vi "Update Scaling Information.vi"(0 "Plugin_UI in":refnum<class "Plugin_UI.lvclass">, 11 "error in (no error)":errorcluster) -> (4 "Plugin_UI out":refnum<class "Plugin_UI.lvclass">, 15 "error out":errorcluster)   [LabVIEW 2020, in "Plugin.lvlib" / "Plugin_UI.lvclass"]
doc: "When the plugin is activated, read the latest scaling information from Module configuration and update it in the corresponding Channel object."
uses:
  Plugin_UI.lvclass
  C:/SVN_LabSys/labsys_lvcode/LabSys_SourceCode/builds/Libraries/LabSys Framework.lvlibp/Configurable Data Node/Configuration Interface/Configuration Interface.lvclass
  Plugin_UI.lvclass/Plugin_UI.ctl
  Read Input Channels[].vi
  Write Input Channels[].vi
  Channels/Input Channels/Input Channels.lvclass
  C:/SVN_LabSys/labsys_lvcode/LabSys_SourceCode/Plugin Template/Source/Code/Channels/Plugin_Channels.lvclass
  builds/Libraries/LabSys Framework.lvlibp/Configurable Data Node/Configuration Interface/Read Module Configuration.vi
  builds/Libraries/LabSys Framework.lvlibp/Configuration Storage/Module Configuration/Get Lookup Tables.vi
  builds/Libraries/LabSys Framework.lvlibp/Configuration Storage/Module Configuration/Get Scaling Functions.vi
  Write Lookup Tables.vi
  Write Scaling Functions.vi
  builds/Libraries/LabSys Framework.lvlibp/Configuration Storage/Module Configuration/Module Configuration.lvclass
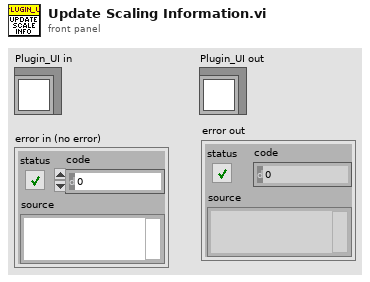
[diagram p1: front panel]
types:
  T1 = typedef "LabSys Framework.lvlibp/Configuration Storage.lvlib/Test Configuration.lvclass/Table Information.ctl" = cluster{"Name":string, "Lookup Table":dbl[][]}
  T2 = typedef "LabSys Framework.lvlibp/Configuration Storage.lvlib/Test Configuration.lvclass/Function Information.ctl" = cluster{"Name":string, "Expression":string, "Constants":T3[], "Test Data":dbl[][]}
  T3 = typedef "LabSys Framework.lvlibp/Configuration Storage.lvlib/Test Configuration.lvclass/Function Constant Value.ctl" = cluster{"Constant Name":string, "Value":dbl}
  T4 = typedef "LabSys Framework.lvlibp/Configuration Storage.lvlib/Test Configuration.lvclass/Channel Information.ctl" = cluster{"Channel Direction":T5, "Alias":string, "Refresh (ms)":dbl, "Scaling Information":T6, "Value Type":T8, "Subchannels":T9[], "Auxiliary Data":variant, "Group":i32}
  T5 = typedef "LabSys Framework.lvlibp/Configuration Storage.lvlib/Test Configuration.lvclass/Channel Directions.ctl" = enum8{"Module Input", "Module Output"}
  T6 = typedef "LabSys Framework.lvlibp/Configuration Storage.lvlib/Test Configuration.lvclass/Scaling Information.ctl" = cluster{"Active":bool, "Scaling Type":T7, "Output Minimum":dbl, "Output Maximum":dbl, "Raw Minimum":dbl, "Raw Maximum":dbl, "Output Unit":string, "Function":string, "Lookup Table":string}
  T7 = typedef "LabSys Framework.lvlibp/Configuration Storage.lvlib/Test Configuration.lvclass/Scaling Types.ctl" = enum8{"Linear", "Function", "Lookup Table"}
  T8 = typedef "Framework Base Library.lvlibp/Value Types.ctl" = enum8{"Unknown", "double", "double array", "Waveform", "DigWaveform", "Boolean", "Decimal", "String", "Db2Message", "Byte Array", "Unsigned Decimal"}
  T9 = typedef "LabSys Framework.lvlibp/Configuration Storage.lvlib/Test Configuration.lvclass/Subchannel Information.ctl" = cluster{"Alias":string, "Start Bit":u32, "Bit Length":u32, "Value Type":T8, "Auxiliary Data":variant}
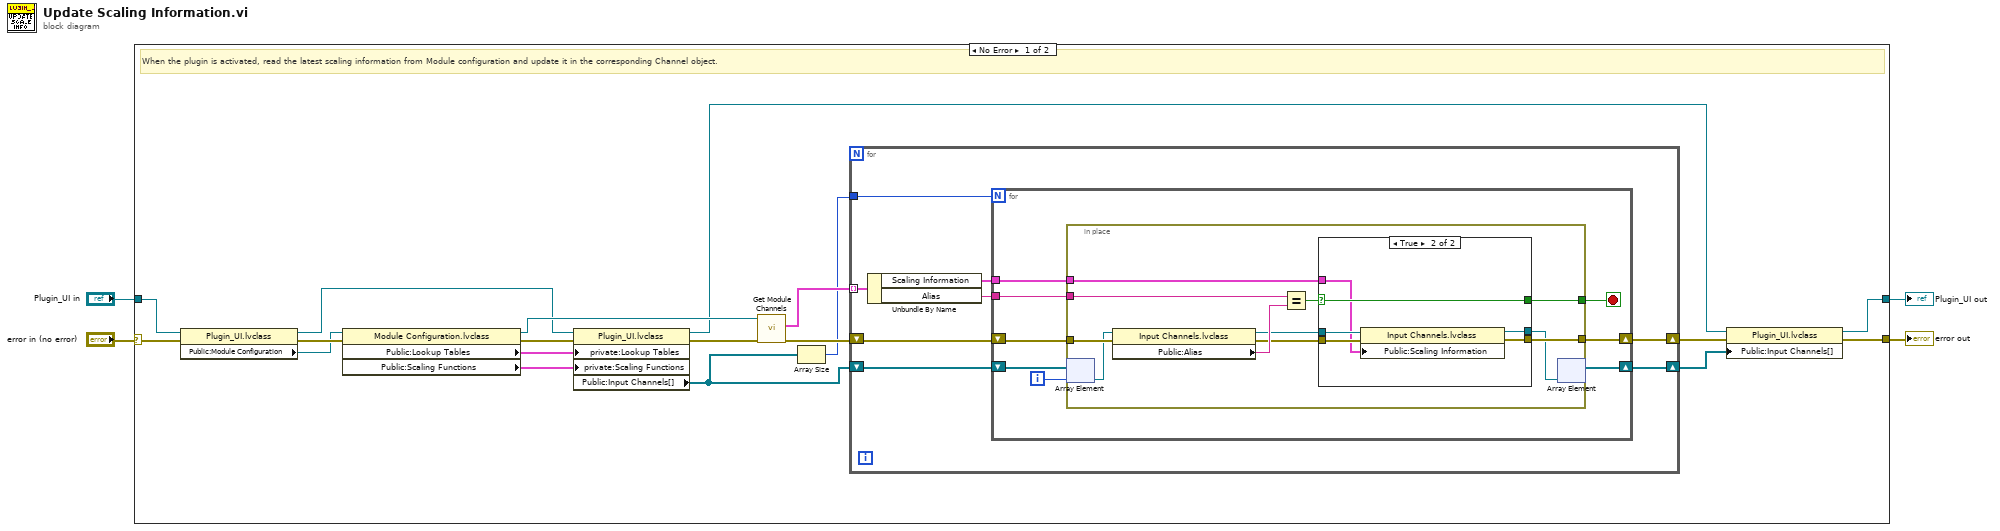
[diagram p0: block diagram]
diagram:
  n1 = case shown="No Error" "error in (no error)" {
    selector: "error in (no error)" -> [w15 w61]
    tunnel: "Plugin_UI in" -> [w21 w60]
    tunnel: [w19 w61] -> w3
    tunnel: [w17 w60] -> w2
    frame No Error {
      # "When the plugin is activated, read the latest scaling information from Module configuration and update it in the corresponding Channel object."
      n2 = property class="Plugin_UI.lvclass"(reference=w21, error in=w15) -> (reference out=w11:refnum<class "Plugin_UI.lvclass">, error out=w14:errorcluster, "Public:Module Configuration"=w13:refnum<class "Module Configuration.lvclass">)
      n3 = property class="Module Configuration.lvclass"(reference=w13, error in=w14) -> (reference out=w12:refnum<class "Module Configuration.lvclass">, error out=w10:errorcluster, "Public:Lookup Tables"=w7:T1[], "Public:Scaling Functions"=w6:T2[])
      n4 = property class="Plugin_UI.lvclass"(reference=w11, error in=w10, "private:Lookup Tables"=w7, "private:Scaling Functions"=w6) -> (reference out=w8:refnum<class "Plugin_UI.lvclass">, error out=w9:errorcluster, "Public:Input Channels[]"=w5:refnum<class "Input Channels.lvclass">[])
      n5 = call-dynamic "Get Module Channels.vi"("error in (no error)"=w9, "Module Configuration in"=w12) -> ("error out"=w23:errorcluster, "Channel Information"=w22:T4[])  [unwired: 7 in, 1 out]
      n6 = Array Size(array=w5) -> (size(s)=w16:i32)
      n7 = for {
        tunnel: w22 -> [w31] mode=indexing
        shift-right: [w27] -> w20
        shift-left: w23 -> [w29]
        shift-right: [w26] -> w18
        shift-left: w5 -> [w30]
        tunnel: w16 -> [w24]
        n8 = Unbundle By Name(w31) -> ("Scaling Information"=w25:T6, "Alias"=w28:string)
        n9 = for {
          N: w24 -> [_]
          tunnel: w28 -> [w38]
          shift-right: [w37] -> w27
          shift-left: w29 -> [w39]
          shift-right: [w34] -> w26
          shift-left: w30 -> [w36]
          tunnel: w25 -> [w32]
          i -> [w35]
          stop <- w33 stop-if-true
          n10 = in-place {
            in-place-border: w39 -> [w50]
            in-place-border: w38 -> [w49]
            in-place-border: [w45] -> w37
            in-place-border: [w41] -> w33
            in-place-border: w32 -> [w40]
            n11 = in-place-array #1(w36, w35) -> (w43:refnum<class "Input Channels.lvclass">)
            n12 = property class="Input Channels.lvclass"(reference=w43, error in=w50) -> (reference out=w46:refnum<class "Input Channels.lvclass">, error out=w47:errorcluster, "Public:Alias"=w48:string)
            n13 = Equal?(x=w49, y=w48) -> (x = y?=w44:bool)
            n14 = case shown="True" w44 {
              selector: w44 -> [w51 w55]
              tunnel: w47 -> [w53 w59]
              tunnel: w46 -> [w52 w58]
              tunnel: [w53 w57] -> w45
              tunnel: [w52 w56] -> w42
              tunnel: [w51 w55] -> w41
              tunnel: w40 -> [_ w54]
              frame False {
              }
              frame True {
                n15 = property class="Input Channels.lvclass"(reference=w58, error in=w59, "Public:Scaling Information"=w54) -> (reference out=w56:refnum<class "Input Channels.lvclass">, error out=w57:errorcluster)
              }
            }
            n16 = in-place-array #1(w42) -> (w34:refnum<class "Input Channels.lvclass">[])  [unwired: 1 out]
          }
        }
      }
      n17 = property class="Plugin_UI.lvclass"(reference=w8, error in=w20, "Public:Input Channels[]"=w18) -> (reference out=w17:refnum<class "Plugin_UI.lvclass">, error out=w19:errorcluster)
    }
    frame Error {
    }
  }
  "Plugin_UI out" <- w2
  "error out" <- w3
